vi "Arm Information.vi"(11 "报警":T1) -> (3 "报警信息":string)   [LabVIEW 2011]
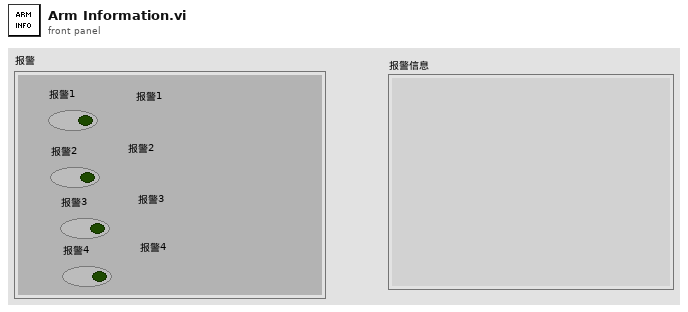
[diagram p1: front panel]
types:
  T1 = cluster{"报警1":bool, "报警2":bool, "报警3":bool, "报警4":bool}
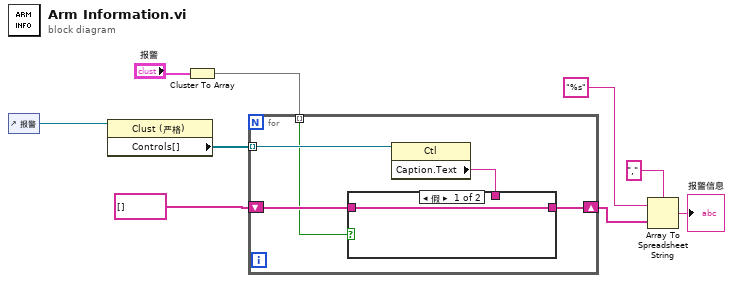
[diagram p0: block diagram]
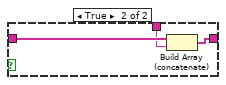
[diagram p2: hidden frame]
diagram:
  n1 = control-ref of="报警"() -> (w9:refnum<vi>)
  n2 = property class="Clust (严格)"(reference=w9) -> ("Controls[]"=w8:refnum<vi>[])  [unwired: 1 in, 2 out]
  n3 = Cluster To Array(cluster="报警") -> (array=w6:bool[])
  n4 = for {
    tunnel: w8 -> [w14] mode=indexing
    tunnel: w6 -> [w11] mode=indexing
    shift-right: [w10] -> w2
    shift-left: string[] [] -> [w12]
    n5 = property class="Ctl"(reference=w14) -> ("Caption.Text"=w13:string)  [unwired: 1 in, 2 out]
    n6 = case shown="假" w11 {
      tunnel: w13 -> [_ w17]
      tunnel: w12 -> [w15 w18]
      tunnel: [w15 w16] -> w10
      frame False {
      }
      frame True {
        n7 = Build Array (concatenate)(w18, w17) -> (w16:string[])
      }
    }
  }
  n8 = Array To Spreadsheet String(delimiter (Tab)="," ("分隔符(Tab)"), array=w2, 3:"%s" ("格式字符串")) -> (spreadsheet string=→"报警信息":string)
